vi "LATP-Server.vi"() -> ()   [LabVIEW 2017]
uses:
  <vilib>/regexp/Match Regular Expression.xnode
  <vilib>/httpClient/LabVIEWHTTPClient.lvlib
panel:
  out "Atmospheric Pressure":dbl
  out "error out":errorcluster
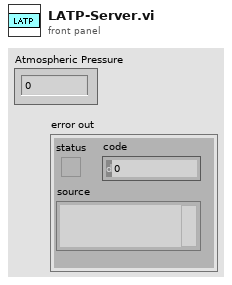
[diagram p1: front panel]
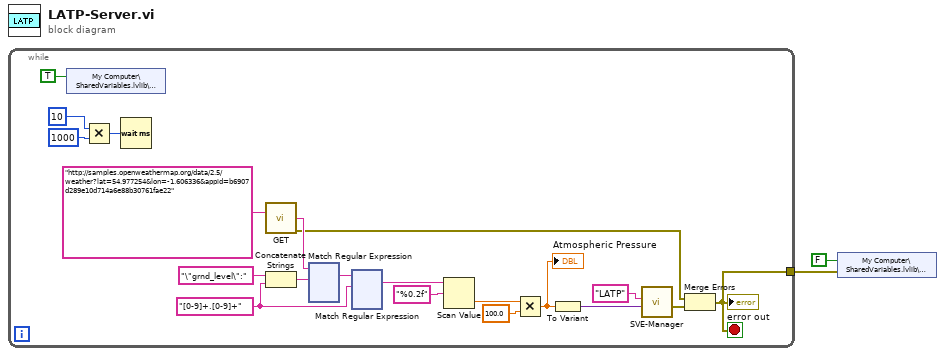
[diagram p0: block diagram]
diagram:
  n1 = while {
    tunnel: [w3] -> w1
    stop <- w3 stop-if-true
    w19 = "[0-9]+.[0-9]+" ("regular expression 2")
    n2 = shared-variable "My Computer\\SharedVariables.lvlib\\LATP-Live"(TRUE ("LATP-Live")) -> ()  [unwired: 1 in, 1 out]
    n3 = Multiply(x=u32 10 ("milliseconds to wait"), y=u32 1000) -> (x*y=w8:u32)
    n4 = Wait (ms)(milliseconds to wait=w8) -> ()  [unwired: 1 out]
    n5 = call <vilib>:"GET.vi"("url"="http://samples.openweathermap.org/data/2.5/weather?lat=54.977254&lon=-1.606336&appid=b6907d289e10d714a6e88b30761fae22") -> ("body"=w13:string, "error out"=w5:errorcluster)  [unwired: 11 in, 2 out]
    n6 = Concatenate Strings("\"grnd_level\":" ("regular expression"), w19) -> (w21:string)
    n7 = xnode "Match Regular Expression"("input string"=w13, "regular expression"=w21) -> ("whole match"=w14:string)  [unwired: 4 in, 4 out]
    n8 = xnode "Match Regular Expression"("input string"=w14, "regular expression"=w19) -> ("whole match"=w15:string)  [unwired: 4 in, 4 out]
    n9 = Scan Value(string=w15, format string="%0.2f") -> (value=w17:dbl)  [unwired: 1 in, 1 out]
    n10 = Multiply(x=w17, y=100.0) -> (x*y=w11:dbl)
    "Atmospheric Pressure" <- w11
    n11 = To Variant(anything=w11) -> (Variant=w10:variant)
    n12 = call "SVE-Manager.vi"("Data"=w10, "DataTag"="LATP") -> ("error out"=w4:errorcluster)  [unwired: 9 in]
    n13 = Merge Errors(w5, w4) -> (w3:errorcluster)
    "error out" <- w3
  }
  n14 = shared-variable "My Computer\\SharedVariables.lvlib\\LATP-Live"(FALSE ("LATP-Live"), error in=w1) -> ()  [unwired: 1 out]
